vi "Set Alias Error.vi"(6 "validation information in":T1, 8 "error in":errorcluster, 10 "alias":T2, 11 "endpoint aliases in":T4 format="%.0x") -> (0 "error out":errorcluster, 1 "veristand error out":errorcluster, 3 "endpoint aliases out":T4 format="%.0x", 4 "validation information out":T1)   [LabVIEW 2017, in "Routing and Faulting Scripting.lvlib"]
uses:
  Routing and Faulting Scripting.lvlib
  <vilib>/NI Veristand/Custom Device API/Custom Device Item Ref.ctl
  Shared/Alias Mapping.ctl
  Shared/Alias Endpoint.ctl
  Validation/Validation Information.ctl
  <vilib>/NI Veristand/Custom Device API/Custom Device API.lvlib
  Shared/Routing and Faulting Shared.lvlib
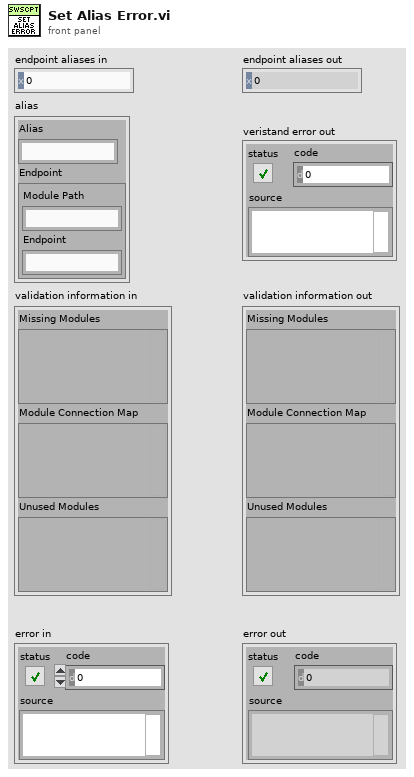
[diagram p1: front panel]
types:
  T1 = typedef "Routing and Faulting Scripting.lvlib/Validation Information.ctl" = cluster{"Missing Modules":variant, "Module Connection Map":variant, "Unused Modules":variant}
  T2 = typedef "Routing and Faulting Shared.lvlib/Alias Mapping.ctl" = cluster{"Alias":string, "Endpoint":T3}
  T3 = typedef "Routing and Faulting Shared.lvlib/Alias Endpoint.ctl" = cluster{"Module Path":string, "Endpoint":string}
  T4 = typedef "Custom Device API.lvlib/Custom Device Item Ref.ctl" = u64
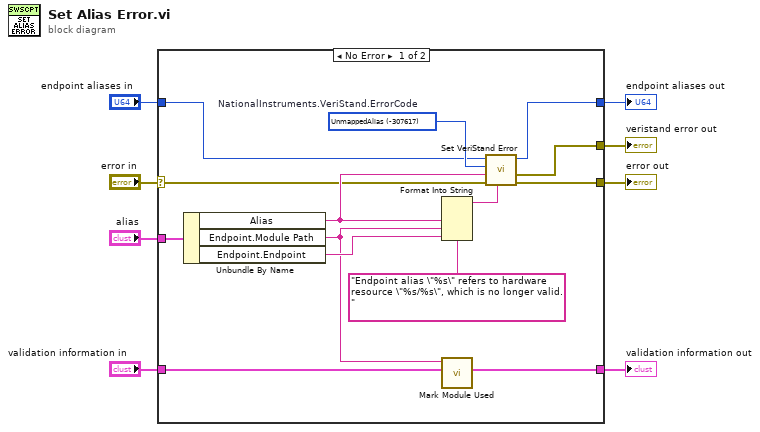
[diagram p0: block diagram]
diagram:
  n1 = case shown="No Error" "error in" {
    selector: "error in" -> [w12 w25]
    tunnel: "endpoint aliases in" -> [w19 w24]
    tunnel: "alias" -> [w18 _]
    tunnel: [w15 w25] -> w6
    tunnel: [w14 w24] -> w5
    tunnel: [w13 _] -> w4
    tunnel: "validation information in" -> [w11 w23]
    tunnel: [w10 w23] -> w1
    frame No Error {
      w22 = -307617 items=["Success"=0, "NoProjectOpen"=-307992, "SequenceCompileError"=-307988, "SessionAlreadyDeployed"=-307984, "SessionNotDeployed"=-307982, "SequenceNotFoundInSession"=-307981, "StimulusProfileSessionLocked"=-307980, "EmptyNodeName"=-307930, "NodeAlreadyExistsByName"=-307926, "NumberOfCoefficientsOutOfRange"=-307884, "DownloadFileError"=-307872, "IncorrectLogFileName"=-307871, "LogTriggerConditionSyntaxError"=-307868, "DuplicateLogSessionName"=-307867, "LogSessionNotFound"=-307865, "ChannelLengthMismatch"=-307830, "NodeNotFoundDuringCompile"=-307829, "ChannelNodeRemoved"=-307828, "NotAChannel"=-307825, "NotAWaveform"=-307824, "STIFileError"=-307784, "DependenciesCycle"=-307783, "ChannelNotFoundInLogFile"=-307782, "ChannelGroupNotFoundInLogFile"=-307781, "GatewayNotOnLocalhost"=-307780, "NotEnoughDynamicDataSharingSpace"=-307738, "TargetMissingDataSharingDevice"=-307737, "ChannelMappingsSizeMismatch"=-307728, "DuplicateChannelAliasMappings"=-307711, "NotAnInlineCustomDevice"=-307710, "IncompatibleModel"=-307703, "ModelDimensionMismatch"=-307702, "SLSCChassisLoadFailed"=-307691, "TargetDisabled"=-307689, "MismatchedLengths"=-307687, "TargetInvalid"=-307686, "ParameterNotFound"=-307685, "ServerPortAlreadyInUse"=-307684, "TargetDisconnected"=-307682, "ServiceConfigurationFile"=-307681, "ModelParameterFileParseError"=-307680, "NoActionRequired"=-307677, "InputParameterInvalid"=-307676, "HostRunningDifferentSystemDefinition"=-307671, "ChannelNotScalable"=-307668, "ChannelCannotBeFaulted"=-307666, "ChannelNotWritable"=-307665, "ChannelNotReadable"=-307664, "Timeout"=-307663, "NodeNotFound"=-307662, "SystemDefinitionDeploymentFailure"=-307661, "SystemDefinitionDeploymentTimeout"=-307660, "EmptyPassword"=-307659, "SystemDefinitionAlreadyActive"=-307658, "InvalidConfigurationPassword"=-307657, "NoSystemDefinitionLoaded"=-307656, "ComponentNotAvailable"=-307655, "NotDeployed"=-307654, "InvalidFile"=-307653, "FailedServerConnection"=-307652, "FunctionNotSupported"=-307651, "UnexpectedError"=-307650, "UnmappedAlias"=-307617, "InvalidStreamConditionForDataType"=-307554, "WaveformDataTypeMismatch"=-307553, "InvalidDaqPluginFile"=-307526, "FileVersionUnsupported"=-307525]  # NationalInstruments.VeriStand.ErrorCode
      n2 = Unbundle By Name(w18) -> ("Alias"=w17:string, "Endpoint.Module Path"=w9:string, "Endpoint.Endpoint"=w16:string)
      n3 = Format Into String(format string="Endpoint alias \"%s\" refers to hardware resource \"%s/%s\", which is no longer valid.", w17, w9, w16) -> (resulting string=w20:string)  [unwired: 2 in, 1 out]
      n4 = call "Mark Module Used.vi"("Validation Information in"=w11, "Module Path"=w9) -> ("Validation Information out"=w10:T1)  [unwired: 8 in, 1 out]
      n5 = call "Set VeriStand Error.vi"("message"=w20, "error in (no error)"=w12, "key"=w17, "errCode"=w22, "Custom Device Item Ref in"=w19) -> ("error out"=w15:errorcluster, "VeriStand Error out"=w13:errorcluster, "Custom Device Item Ref out"=w14:T4)  [unwired: 4 in]
    }
    frame Error {
    }
  }
  "endpoint aliases out" <- w5
  "error out" <- w6
  "veristand error out" <- w4
  "validation information out" <- w1
